vi "Modbus FVIR Sensors.vi"(8 "error in":errorcluster, 11 "PLC Data":T1 {"PLC Data - LDO"."Timing"."Absolute Time" format="%<%H:%M:%S%3u>t"; "PLC Data - LDO"."Timing"."Display Time" format="%#.20f"; "PLC Data - LDO"."Timing"."Test Time Ref" format="%#.20f"; "PLC Data - LDO"."Timing"."Precondition Time Ref" format="%#.20f"; "PLC Data - LDO"."Timing"."First Call Time Ref" format="%#.20f"; "PLC Data - FVIR"."Timing"."Absolute Time" format="%<%H:%M:%S%3u>t"; "PLC Data - FVIR"."Timing"."Display Time" format="%#.20f"; "PLC Data - FVIR"."Timing"."Test Time Ref" format="%#.20f"; "PLC Data - FVIR"."Timing"."Precondition Time Ref" format="%#.20f"; "PLC Data - FVIR"."Timing"."First Call Time Ref" format="%#.20f"}) -> (0 "error out":errorcluster, 3 "PLC Data Out":T1 {"PLC Data - LDO"."Timing"."Absolute Time" format="%<%H:%M:%S%3u>t"; "PLC Data - LDO"."Timing"."Display Time" format="%#.20f"; "PLC Data - LDO"."Timing"."Test Time Ref" format="%#.20f"; "PLC Data - LDO"."Timing"."Precondition Time Ref" format="%#.20f"; "PLC Data - LDO"."Timing"."First Call Time Ref" format="%#.20f"; "PLC Data - FVIR"."Timing"."Absolute Time" format="%<%H:%M:%S%3u>t"; "PLC Data - FVIR"."Timing"."Display Time" format="%#.20f"; "PLC Data - FVIR"."Timing"."Test Time Ref" format="%#.20f"; "PLC Data - FVIR"."Timing"."Precondition Time Ref" format="%#.20f"; "PLC Data - FVIR"."Timing"."First Call Time Ref" format="%#.20f"})   [LabVIEW 2020, in "Modbus.lvlib"]
uses:
  Modbus.lvlib
  Modbus PLC Data All.ctl
  Modbus FVIR Control.ctl
  Modbus Timing.ctl
  <vilib>/Utility/miscctls.llb/LVDateTimeRec.ctl
  Modbus LDO Control.ctl
  WritingDataFile/Data to Save.ctl
  support/Terminate Conditions Cluster.ctl
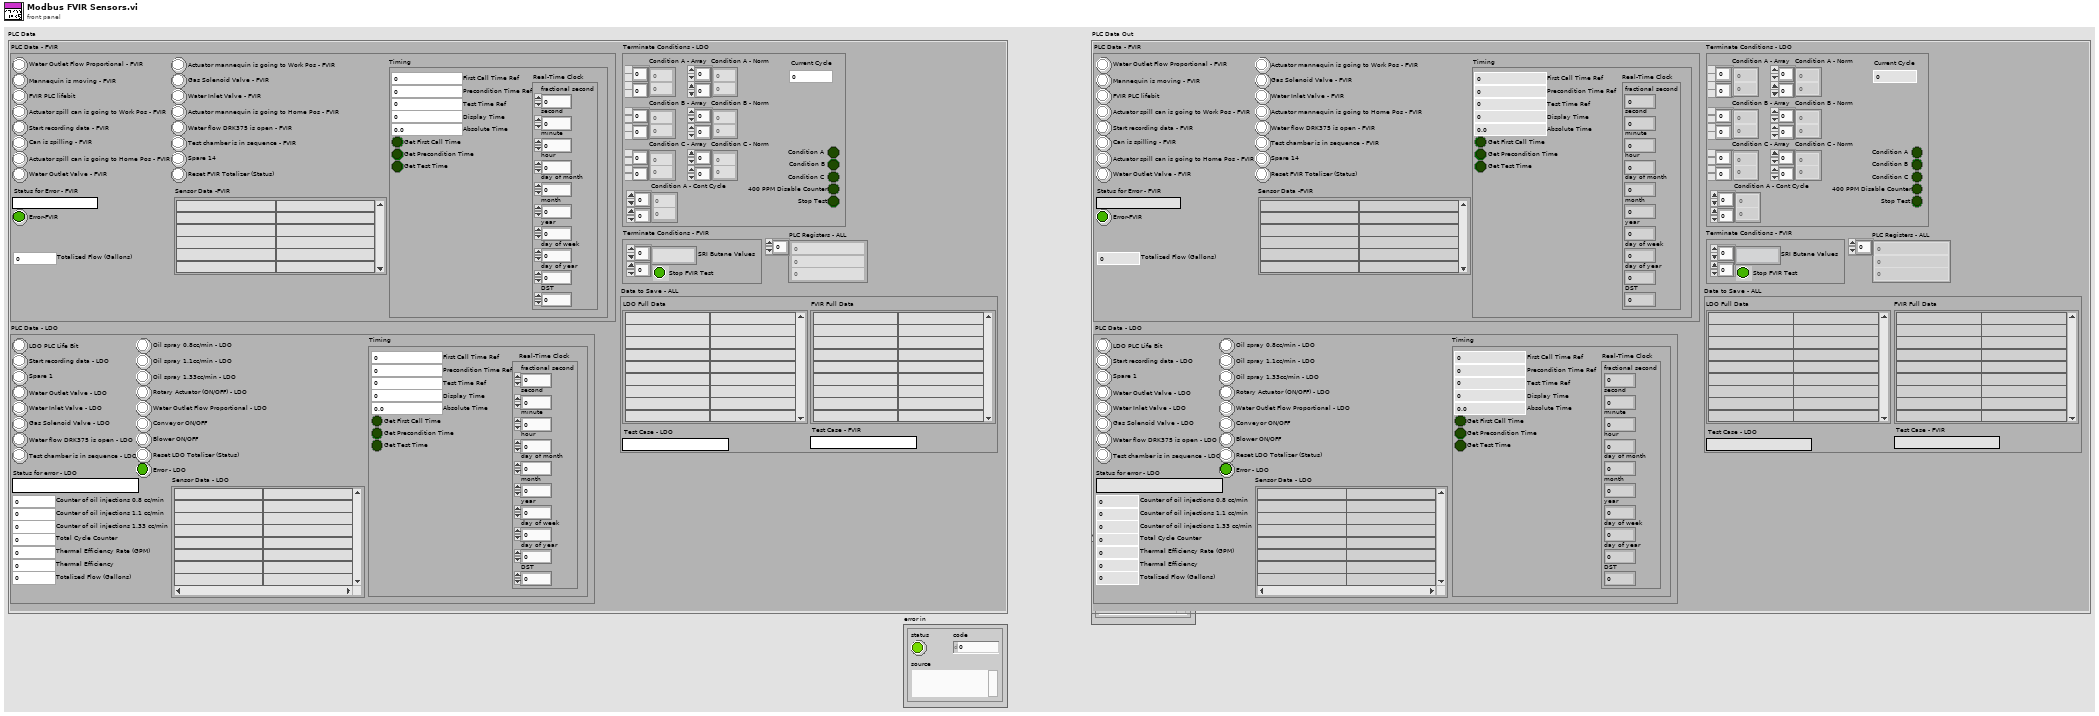
[diagram p1: front panel]
types:
  T1 = typedef "Modbus PLC Data All.ctl" = cluster{"PLC Data - FVIR":T2, "PLC Data - LDO":T5, "PLC Registers - ALL":i16[], "Data to Save - ALL":T6, "Terminate Conditions - LDO":T7, "Terminate Conditions - FVIR":cluster{"SRI Butane Values":string[][], "Stop FVIR Test":bool}}
  T2 = typedef "Modbus FVIR Control.ctl" = cluster{"Reset FVIR Totalizer (Status)":bool, "Spare 14":bool, "Actuator mannequin is going to Work Pos - FVIR":bool, "Actuator mannequin is going to Home Pos - FVIR":bool, "Test chamber is in sequence - FVIR ":bool, "Water flow DRK375 is open - FVIR":bool, "Gas Solenoid Valve - FVIR":bool, "Water Inlet Valve - FVIR":bool, "Water Outlet Flow Proportional - FVIR":bool, "Start recording data - FVIR":bool, "Actuator spill can is going to Work Pos - FVIR":bool, "Actuator spill can is going to Home Pos - FVIR":bool, "Water Outlet Valve - FVIR":bool, "Can is spilling - FVIR":bool, "Mannequin is moving - FVIR":bool, "FVIR PLC lifebit":bool, "Status for Error - FVIR":string, "Error-FVIR":bool, "Sensor Data -FVIR":string[][], "Totalized Flow (Gallons)":dbl, "Timing":T3}
  T3 = typedef "Modbus Timing.ctl" = cluster{"First Call Time Ref":dbl, "Precondition Time Ref":dbl, "Test Time Ref":dbl, "Get First Call Time":bool, "Get Precondition Time":bool, "Get Test Time":bool, "Display Time":dbl, "Real-Time Clock":T4, "Absolute Time":dbl}
  T4 = typedef "LVDateTimeRec.ctl" = cluster{"fractional second":dbl, "second":i32, "minute":i32, "hour":i32, "day of month":i32, "month":i32, "year":i32, "day of week":i32, "day of year":i32, "DST":i32}
  T5 = typedef "Modbus LDO Control.ctl" = cluster{"LDO PLC Life Bit":bool, "Start recording data - LDO":bool, "Spare 1":bool, "Water Outlet Valve - LDO":bool, "Water Inlet Valve - LDO":bool, "Gas Solenoid Valve - LDO":bool, "Water flow DRK375 is open - LDO":bool, "Test chamber is in sequence - LDO":bool, "Oil spray 0.8cc/min - LDO":bool, "Oil spray 1.1cc/min - LDO":bool, "Oil spray 1.33cc/min - LDO":bool, "Rotary Actuator (ON/OFF) - LDO":bool, "Water Outlet Flow Proportional - LDO":bool, "Conveyor ON/OFF":bool, "Blower ON/OFF":bool, "Reset LDO Totalizer (Status)":bool, "Status for error - LDO":string, "Error - LDO":bool, "Sensor Data - LDO":string[][], "Thermal Efficiency Rate (GPM)":dbl, "Thermal Efficiency":dbl, "Totalized Flow (Gallons)":dbl, "Counter of oil injections 1.33 cc/min":u16, "Total Cycle Counter":u16, "Counter of oil injections 1.1 cc/min":u16, "Counter of oil injections 0.8 cc/min":u16, "Timing":T3}
  T6 = typedef "Data to Save.ctl" = cluster{"LDO Full Data":string[][], "FVIR Full Data":string[][], "Test Case - FVIR":string, "Test Case - LDO":string}
  T7 = typedef "Terminate Conditions Cluster.ctl" = cluster{"Condition B - Array":dbl[][], "Current Cycle":u16, "Condition C - Array":dbl[][], "Condition A - Array":dbl[][], "400 PPM Disable Counter":bool, "Condition A - Norm":dbl[][], "Condition B - Norm":dbl[][], "Condition C - Norm":dbl[][], "Condition A":bool, "Condition B":bool, "Condition C":bool, "Condition A - Cont Cycle":dbl[][], "Stop Test":bool}
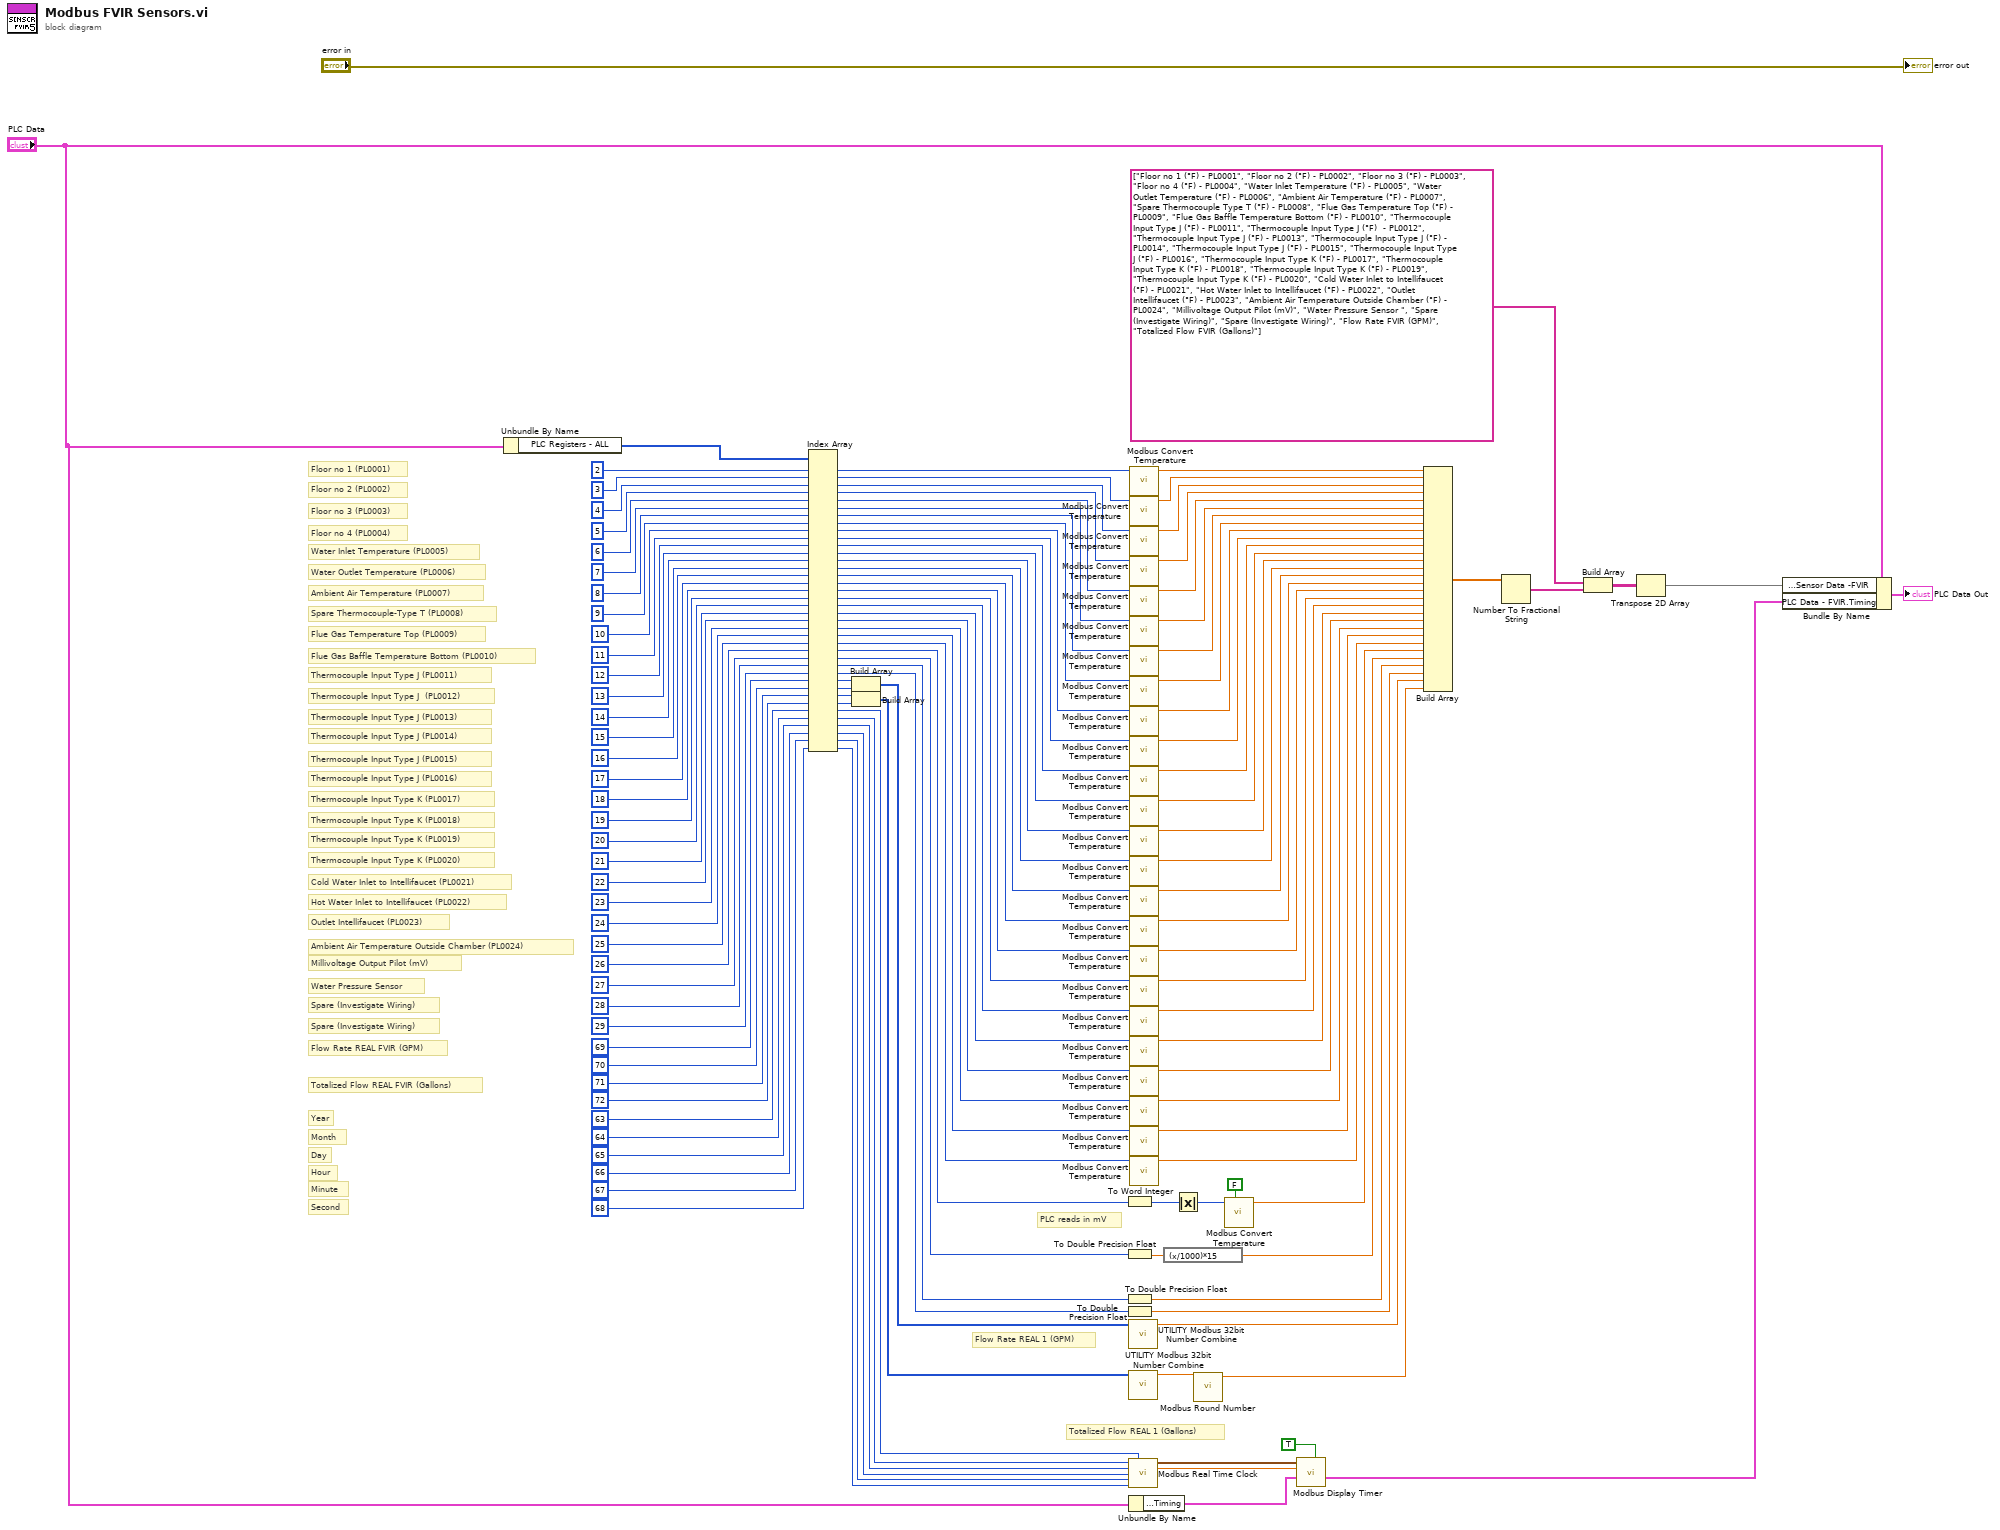
[diagram p0: block diagram]
diagram:
  # "PLC reads in mV"
  # "Second"
  # "Minute"
  # "Hour"
  # "Day"
  # "Month"
  # "Year"
  # "Totalized Flow REAL FVIR (Gallons)"
  # "Flow Rate REAL FVIR (GPM)"
  # "Totalized Flow REAL 1 (Gallons)"
  # "Flow Rate REAL 1 (GPM)"
  # "Spare (Investigate Wiring)"
  # "Spare (Investigate Wiring)"
  # "Water Pressure Sensor"
  # "Millivoltage Output Pilot (mV)"
  # "Ambient Air Temperature Outside Chamber (PL0024)"
  # "Outlet Intellifaucet (PL0023)"
  # "Hot Water Inlet to Intellifaucet (PL0022)"
  # "Cold Water Inlet to Intellifaucet (PL0021)"
  # "Thermocouple Input Type K (PL0020)"
  # "Thermocouple Input Type K (PL0019)"
  # "Thermocouple Input Type K (PL0018)"
  # "Thermocouple Input Type K (PL0017)"
  # "Thermocouple Input Type J (PL0016)"
  # "Thermocouple Input Type J (PL0015)"
  # "Thermocouple Input Type J (PL0014)"
  # "Thermocouple Input Type J (PL0013)"
  # "Thermocouple Input Type J  (PL0012)"
  # "Thermocouple Input Type J (PL0011)"
  # "Flue Gas Baffle Temperature Bottom (PL0010)"
  # "Flue Gas Temperature Top (PL0009)"
  # "Spare Thermocouple-Type T (PL0008)"
  # "Ambient Air Temperature (PL0007)"
  # "Water Outlet Temperature (PL0006)"
  # "Water Inlet Temperature (PL0005)"
  # "Floor no 4 (PL0004)"
  # "Floor no 3 (PL0003)"
  # "Floor no 2 (PL0002)"
  # "Floor no 1 (PL0001)"
  n1 = Unbundle By Name("PLC Data") -> ("PLC Registers - ALL"=w41:i16[])
  n2 = Index Array(array=w41, index #1=2 ("index"), index #2=3 ("index"), index #3=4 ("index"), index #4=5 ("index"), index #5=6 ("index"), index #6=7 ("index"), index #7=8 ("index"), index #8=9 ("index"), index #9=10 ("index"), index #10=11 ("index"), index #11=12 ("index"), index #12=13 ("index"), index #13=14 ("index"), index #14=15 ("index"), index #15=16 ("index"), index #16=17 ("index"), index #17=18 ("index"), index #18=19 ("index"), index #19=20 ("index"), index #20=21 ("index"), index #21=22 ("index"), index #22=23 ("index"), index #23=24 ("index"), index #24=25 ("index"), index #25=26 ("index"), index #26=27 ("index"), index #27=28 ("index"), index #28=29 ("index"), index #29=69 ("index"), index #30=70 ("index"), index #31=71 ("index"), index #32=72 ("index"), index #33=63 ("index"), index #34=64 ("index"), index #35=65 ("index"), index #36=66 ("index"), index #37=67 ("index"), index #38=68 ("index")) -> (element #1=w98:i16, element #2=w97:i16, element #3=w96:i16, element #4=w95:i16, element #5=w94:i16, element #6=w93:i16, element #7=w92:i16, element #8=w91:i16, element #9=w90:i16, element #10=w89:i16, element #11=w88:i16, element #12=w87:i16, element #13=w86:i16, element #14=w85:i16, element #15=w84:i16, element #16=w83:i16, element #17=w82:i16, element #18=w81:i16, element #19=w80:i16, element #20=w79:i16, element #21=w78:i16, element #22=w77:i16, element #23=w76:i16, element #24=w75:i16, element #25=w3:i16, element #26=w8:i16, element #27=w48:i16, element #28=w50:i16, element #29=w30:i16, element #30=w29:i16, element #31=w28:i16, element #32=w27:i16, element #33=w20:i16, element #34=w19:i16, element #35=w18:i16, element #36=w17:i16, element #37=w16:i16, element #38=w15:i16)
  n3 = Build Array(w30, w29) -> (w39:i16[])
  n4 = Build Array(w28, w27) -> (w38:i16[])
  n5 = To Word Integer(number=w3) -> (16bit integer=w5:i16)
  n6 = To Double Precision Float(number=w8) -> (double precision float=w1:dbl)
  n7 = To Double Precision Float(number=w48) -> (double precision float=w47:dbl)
  n8 = To Double Precision Float(number=w50) -> (double precision float=w49:dbl)
  n9 = call "UTILITY Modbus 32bit Number Combine.vi"("Holding Registers"=w39) -> ("Data"=w36:sgl)  [unwired: 9 in, 1 out]
  n10 = call "UTILITY Modbus 32bit Number Combine.vi"("Holding Registers"=w38) -> ("Data"=w37:sgl)  [unwired: 9 in, 1 out]
  n11 = call "Modbus Real Time Clock.vi"("Month"=w19, "Year"=w20, "Day"=w18, "Hour"=w17, "Minute"=w16, "Second"=w15) -> ("Real-Time Clock"=w13:T4, "Absolute Time"=w12:dbl)  [unwired: 8 in]
  n12 = Unbundle By Name("PLC Data") -> ("PLC Data - FVIR.Timing"=w10:T3)
  n13 = call "Modbus Convert Temperature.vi"("PLC Value"=w98) -> ("Converted Value"=w74:dbl)  [unwired: 9 in, 1 out]
  n14 = call "Modbus Convert Temperature.vi"("PLC Value"=w97) -> ("Converted Value"=w73:dbl)  [unwired: 9 in, 1 out]
  n15 = call "Modbus Convert Temperature.vi"("PLC Value"=w96) -> ("Converted Value"=w72:dbl)  [unwired: 9 in, 1 out]
  n16 = call "Modbus Convert Temperature.vi"("PLC Value"=w95) -> ("Converted Value"=w71:dbl)  [unwired: 9 in, 1 out]
  n17 = call "Modbus Convert Temperature.vi"("PLC Value"=w94) -> ("Converted Value"=w70:dbl)  [unwired: 9 in, 1 out]
  n18 = call "Modbus Convert Temperature.vi"("PLC Value"=w93) -> ("Converted Value"=w69:dbl)  [unwired: 9 in, 1 out]
  n19 = call "Modbus Convert Temperature.vi"("PLC Value"=w92) -> ("Converted Value"=w68:dbl)  [unwired: 9 in, 1 out]
  n20 = call "Modbus Convert Temperature.vi"("PLC Value"=w91) -> ("Converted Value"=w67:dbl)  [unwired: 9 in, 1 out]
  n21 = call "Modbus Convert Temperature.vi"("PLC Value"=w90) -> ("Converted Value"=w66:dbl)  [unwired: 9 in, 1 out]
  n22 = call "Modbus Convert Temperature.vi"("PLC Value"=w89) -> ("Converted Value"=w65:dbl)  [unwired: 9 in, 1 out]
  n23 = call "Modbus Convert Temperature.vi"("PLC Value"=w88) -> ("Converted Value"=w64:dbl)  [unwired: 9 in, 1 out]
  n24 = call "Modbus Convert Temperature.vi"("PLC Value"=w87) -> ("Converted Value"=w63:dbl)  [unwired: 9 in, 1 out]
  n25 = call "Modbus Convert Temperature.vi"("PLC Value"=w86) -> ("Converted Value"=w62:dbl)  [unwired: 9 in, 1 out]
  n26 = call "Modbus Convert Temperature.vi"("PLC Value"=w85) -> ("Converted Value"=w61:dbl)  [unwired: 9 in, 1 out]
  n27 = call "Modbus Convert Temperature.vi"("PLC Value"=w84) -> ("Converted Value"=w60:dbl)  [unwired: 9 in, 1 out]
  n28 = call "Modbus Convert Temperature.vi"("PLC Value"=w83) -> ("Converted Value"=w59:dbl)  [unwired: 9 in, 1 out]
  n29 = call "Modbus Convert Temperature.vi"("PLC Value"=w82) -> ("Converted Value"=w58:dbl)  [unwired: 9 in, 1 out]
  n30 = call "Modbus Convert Temperature.vi"("PLC Value"=w81) -> ("Converted Value"=w57:dbl)  [unwired: 9 in, 1 out]
  n31 = call "Modbus Convert Temperature.vi"("PLC Value"=w80) -> ("Converted Value"=w56:dbl)  [unwired: 9 in, 1 out]
  n32 = call "Modbus Convert Temperature.vi"("PLC Value"=w79) -> ("Converted Value"=w55:dbl)  [unwired: 9 in, 1 out]
  n33 = call "Modbus Convert Temperature.vi"("PLC Value"=w78) -> ("Converted Value"=w54:dbl)  [unwired: 9 in, 1 out]
  n34 = call "Modbus Convert Temperature.vi"("PLC Value"=w77) -> ("Converted Value"=w53:dbl)  [unwired: 9 in, 1 out]
  n35 = call "Modbus Convert Temperature.vi"("PLC Value"=w76) -> ("Converted Value"=w52:dbl)  [unwired: 9 in, 1 out]
  n36 = call "Modbus Convert Temperature.vi"("PLC Value"=w75) -> ("Converted Value"=w51:dbl)  [unwired: 9 in, 1 out]
  n37 = expression code="(x/1000)*15"(w1) -> (w7:dbl)
  n38 = Absolute Value(x=w5) -> (abs(x)=w6:i16)
  n39 = call "Modbus Round Number.vi"("Number"=w37) -> ("Rounded Number"=w35:dbl)  [unwired: 10 in]
  n40 = call "Modbus Convert Temperature.vi"("Divide by 100?"=FALSE, "PLC Value"=w6) -> ("Converted Value"=w2:dbl)  [unwired: 8 in, 1 out]
  n41 = call "Modbus Display Timer.vi"("FVIR?"=TRUE, "Timing in"=w10, "Absolute Time"=w12, "Real-Time Clock"=w13) -> ("Timing Out"=w9:T3)  [unwired: 7 in]
  n42 = Build Array(w74, w73, w72, w71, w70, w69, w68, w67, w66, w65, w64, w63, w62, w61, w60, w59, w58, w57, w56, w55, w54, w53, w52, w51, w2, w7, w47, w49, w36, w35) -> (w44:dbl[])
  n43 = Number To Fractional String(number=w44) -> (F-format string=w45:string[])  [unwired: 3 in]
  n44 = Build Array(string[] ["Floor no 1 (°F) - PL0001", "Floor no 2 (°F) - PL0002", "Floor no 3 (°F) - PL0003", "Floor no 4 (°F) - PL0004", "Water Inlet Temperature (°F) - PL0005", "Water Outlet Temperature (°F) - PL0006", "Ambient Air Temperature (°F) - PL0007", "Spare Thermocouple Type T (°F) - PL0008", "Flue Gas Temperature Top (°F) - PL0009", "Flue Gas Baffle Temperature Bottom (°F) - PL0010", "Thermocouple Input Type J (°F) - PL0011", "Thermocouple Input Type J (°F)  - PL0012", "Thermocouple Input Type J (°F) - PL0013", "Thermocouple Input Type J (°F) - PL0014", "Thermocouple Input Type J (°F) - PL0015", "Thermocouple Input Type J (°F) - PL0016", "Thermocouple Input Type K (°F) - PL0017", "Thermocouple Input Type K (°F) - PL0018", "Thermocouple Input Type K (°F) - PL0019", "Thermocouple Input Type K (°F) - PL0020", "Cold Water Inlet to Intellifaucet (°F) - PL0021", "Hot Water Inlet to Intellifaucet (°F) - PL0022", "Outlet Intellifaucet (°F) - PL0023", "Ambient Air Temperature Outside Chamber (°F) - PL0024", "Millivoltage Output Pilot (mV)", "Water Pressure Sensor ", "Spare (Investigate Wiring)", "Spare (Investigate Wiring)", "Flow Rate FVIR (GPM)", "Totalized Flow FVIR (Gallons)"], w45) -> (w46:string[][])
  n45 = Transpose 2D Array(2D array=w46) -> (transposed array=w42:string[][])
  n46 = Bundle By Name(cluster="PLC Data", "PLC Data - FVIR.Sensor Data -FVIR"=w42, "PLC Data - FVIR.Timing"=w9) -> (→"PLC Data Out":T1)
  "error out" <- "error in"
